vi "WriteSizeNchwMat_SGL.vi"(4 "Width":i32, 6 "Height":i32, 8 "error in":errorcluster, 9 "Channels":i32, 10 "Dimensions":i32, 11 "Array":sgl[][][][](array[numeric])) -> (0 "error out":errorcluster, 3 "Array":sgl[][][][](array[numeric]))   [LabVIEW 2020, in "OpenLvVision_OpenCv.lvlib"]
uses:
  OpenLvVision_OpenCv.lvlib
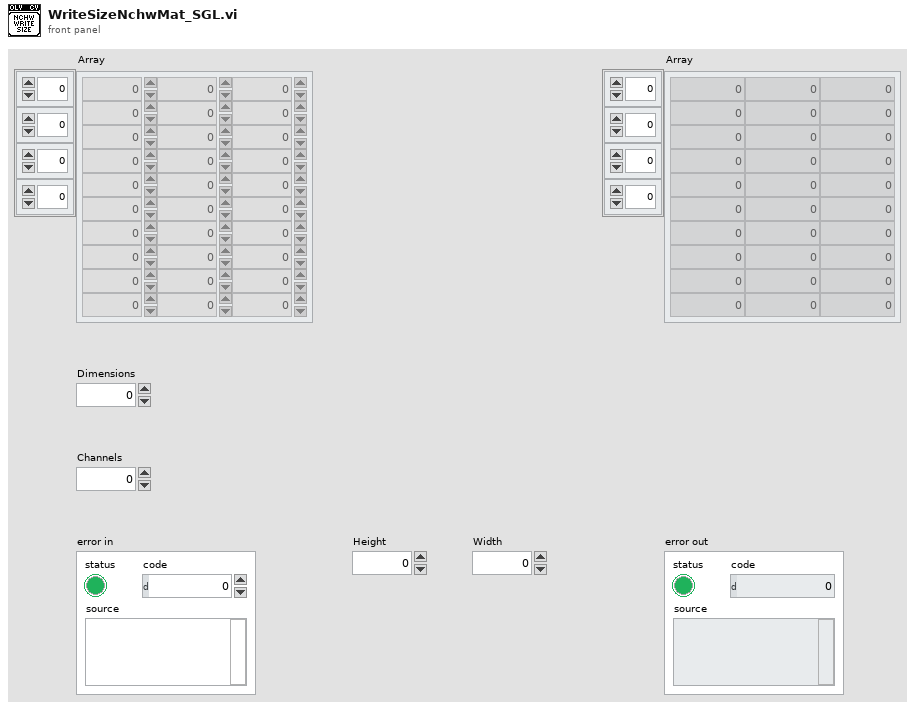
[diagram p1: front panel]
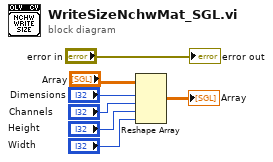
[diagram p0: block diagram]
diagram:
  n1 = Reshape Array("Array", "Dimensions", "Channels", "Height", "Width") -> (→"Array":sgl[][][][])
  "error out" <- "error in"
